vi "example_llm_ollama_unit_test_1.vi"() -> ()   [LabVIEW 2020]
uses:
  src/models/llm_ollama_chatmodels/llm_ollama_chatmodels.lvclass
  src/models/message_text/message_text.lvclass
  D:/lv_llm/labview-llm-libraries/src/models/abstract_message_base/abstract_message_base.lvclass
  src/models/message_text/message.ctl
panel:
  in  "Ollama URL":string="http://localhost:11434/"
  in  "Messages":cluster{"role":string, "text":string}[](array[cluster])=[{"role"="system", "text"="Act as a math teacher and guide the student in solving the problem. You should not solve the problem. Always answer in single line."}, {"role"="user", "text"="What is x in the equation 2x + 3 = 5  ?"}]
  out "error out":errorcluster
  in  "model_name":string(combo)="llama3.1"
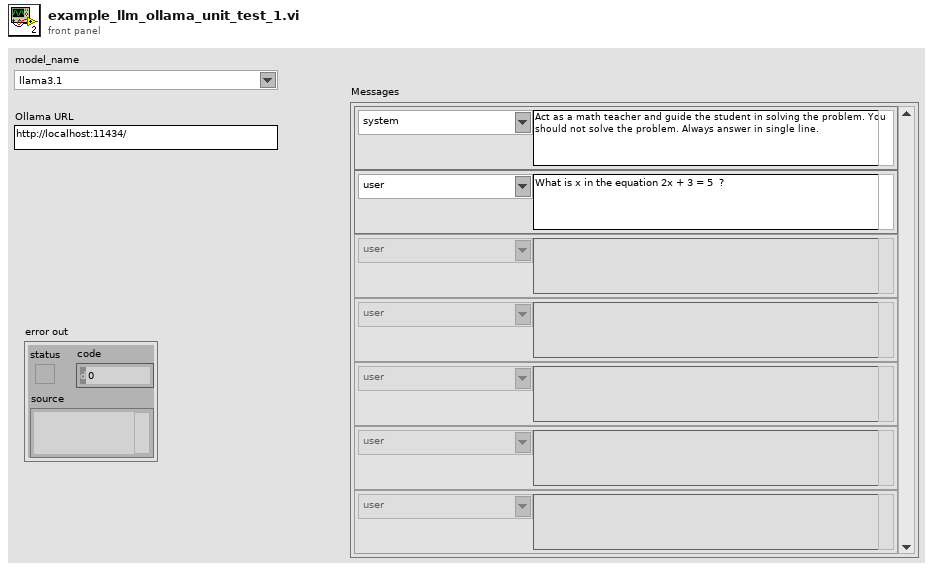
[diagram p1: front panel]
types:
  T1 = typedef "message_text.lvclass/message.ctl" = cluster{"role":string, "content":string[]}
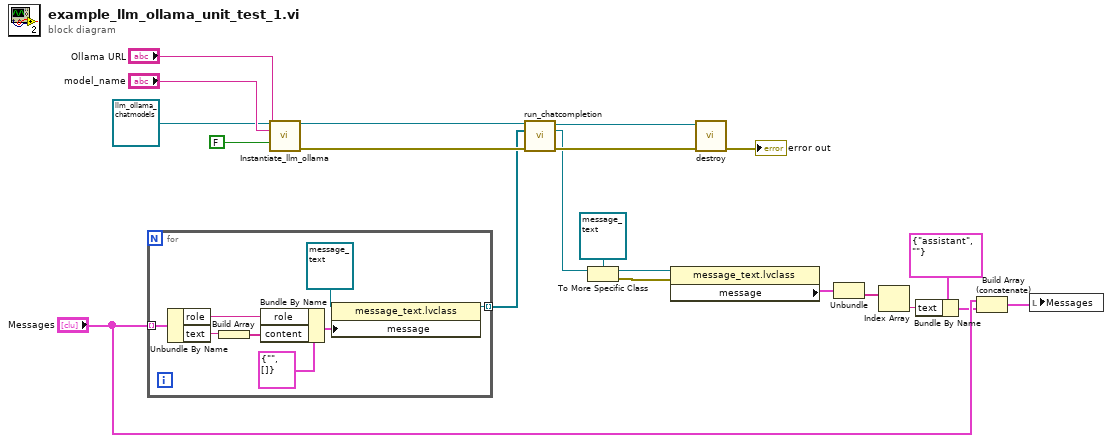
[diagram p0: block diagram]
diagram:
  n1 = for {
    tunnel: "Messages" -> [w27] mode=indexing
    tunnel: [w28] -> w15 mode=indexing
    n2 = Unbundle By Name(w27) -> ("role"=w25:string, "text"=w23:string)
    n3 = Build Array(w23) -> (w22:string[])
    n4 = Bundle By Name(cluster=T1 {"role"="", "content"=[]} ("message"), "role"=w25, "content"=w22) -> (w24:T1)
    n5 = property class="message_text.lvclass"(reference=refnum<class "message_text.lvclass"> refnum ("message_text.lvclass"), "message"=w24) -> (reference out=w28:refnum<class "message_text.lvclass">)  [unwired: 1 in, 1 out]
  }
  n6 = call "Instantiate_llm_ollama.vi"("llm_ollama_chatmodels in"=refnum<class "llm_ollama_chatmodels.lvclass"> refnum ("llm_ollama_chatmodels.lvclass"), "model_name"="model_name", "Ollama URL"="Ollama URL", "EnableStreaming"=FALSE) -> ("llm_ollama_chatmodels out"=w21:refnum<class "llm_ollama_chatmodels.lvclass">, "error out"=w20:errorcluster)  [unwired: 10 in]
  n7 = call-dynamic "run_chatcompletion.vi"("llm_ollama_chatmodels in"=w21, "Messages"=w15, "error in (no error)"=w20) -> ("llm_ollama_chatmodels out"=w18:refnum<class "llm_ollama_chatmodels.lvclass">, "Response"=w3:refnum<class "abstract_message_base.lvclass">, "error out"=w17:errorcluster)  [unwired: 10 in]
  n8 = To More Specific Class(target class=refnum<class "message_text.lvclass"> refnum ("message_text.lvclass"), reference=w3) -> (specific class reference=w1:refnum<class "message_text.lvclass">, error out=w4:errorcluster)  [unwired: 1 in]
  n9 = property class="message_text.lvclass"(reference=w1, error in=w4) -> ("message"=w7:T1)  [unwired: 2 out]
  n10 = call-dynamic "destroy.vi"("error in (no error)"=w17, "abstract_llm_base in"=w18) -> ("error out"=→"error out":errorcluster)  [unwired: 8 in, 1 out]
  n11 = Unbundle(w7) -> ("content"=w6:string[])  [unwired: 1 out]
  n12 = Index Array(array=w6) -> (element=w5:string)  [unwired: 1 in]
  n13 = Bundle By Name(cluster=cluster{"role":string, "text":string} {"role"="assistant", "text"=""} ("message"), "text"=w5) -> (w11:cluster{"role":string, "text":string})
  n14 = Build Array (concatenate)("Messages", w11) -> (w13:cluster{"role":string, "text":string}[])
  n15 = local write "Messages"(w13) -> ()
